vi "PH_BeamlineInformation.Efficiency Calculator.vi"(1 "Later Subystem":dbl, 2 "Former Subsystem":dbl) -> (0 "Efficiency Factor":dbl format="%#_3p")   [LabVIEW 2014, in "PH_BeamlineInformation.lvlib"]
uses:
  PH_BeamlineInformation.lvlib
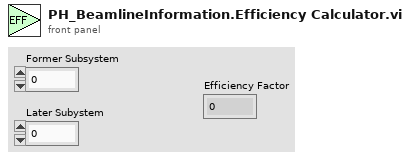
[diagram p1: front panel]
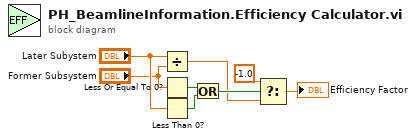
[diagram p0: block diagram]
diagram:
  n1 = Divide(x="Later Subystem", y="Former Subsystem") -> (x/y=w2:dbl)
  n2 = Less Or Equal To 0?(x="Former Subsystem") -> (x <= 0?=w7:bool)
  n3 = Less Than 0?(x="Later Subystem") -> (x < 0?=w6:bool)
  n4 = Or(x=w7, y=w6) -> (x .or. y?=w4:bool)
  n5 = Select(t=-1.0 ("f"), s=w4, f=w2) -> (s? t:f=→"Efficiency Factor":dbl)
